vi "Calculate pulse train duration.vi"(9 "Pulse width (ticks)":u32, 11 "Channel timings in (ticks)":u32[](array[numeric])=[0, 0, 0, 0]) -> (0 "Channel timings out (ticks)":u32[](array[numeric]), 3 "Pulse train length (ticks) out":u32)   [LabVIEW 2013]
doc: "The pulse train duration is the highest channel timing in ticks + the pulse width in ticks."
panel:
  # "Calculate pulse train duration"
  # "The pulse train duration is the highest channel timing in ticks + the pulse width in ticks."
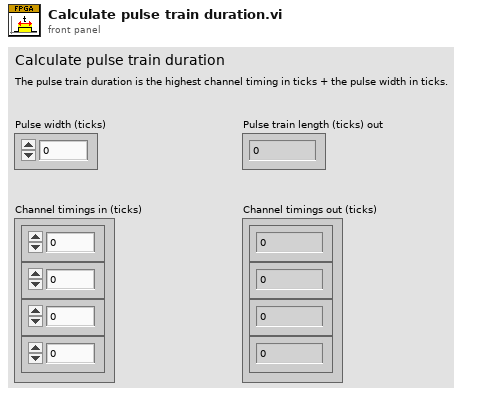
[diagram p1: front panel]
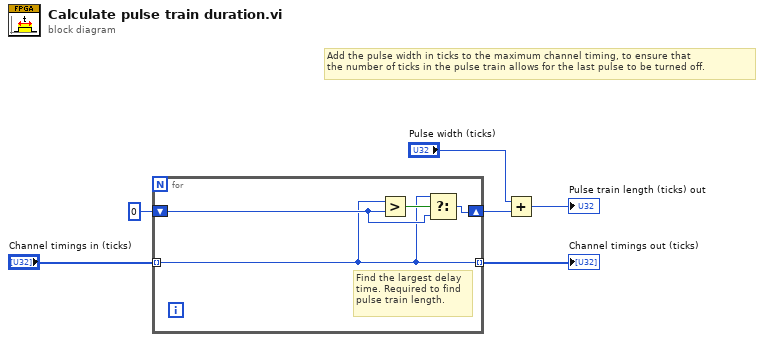
[diagram p0: block diagram]
diagram:
  # "Add the pulse width in ticks to the maximum channel timing, to ensure that\nthe number of ticks in the pulse train allows for the last pulse to be turned off."
  n1 = for {
    tunnel: [w7] -> w6 mode=indexing
    shift-right: [w10] -> w2
    shift-left: u32 0 -> [w8]
    tunnel: "Channel timings in (ticks)" -> [w7] mode=indexing
    # "Find the largest delay\ntime. Required to find\npulse train length."
    n2 = Greater?(x=w7, y=w8) -> (0:w9:bool)
    n3 = Select(t=w7, s=w9, f=w8) -> (s? t:f=w10:u32)
  }
  "Channel timings out (ticks)" <- w6
  n4 = Add(x="Pulse width (ticks)", y=w2) -> (x+y=→"Pulse train length (ticks) out":u32)
